vi "Facade_Create.vi"(0 "reference in":refnum<class "Facade.lvclass">, 2 "Home":refnum<class "House.lvclass">, 5 "Error In":errorcluster) -> (14 "reference out":refnum<class "Facade.lvclass">, 19 "Error Out":errorcluster)   [LabVIEW 2024, in "Facade.lvclass"]
uses:
  Facade.lvclass
  Facade.lvclass/Facade.ctl
  House/House_class/House.lvclass
panel:
  # "Connector Pane"
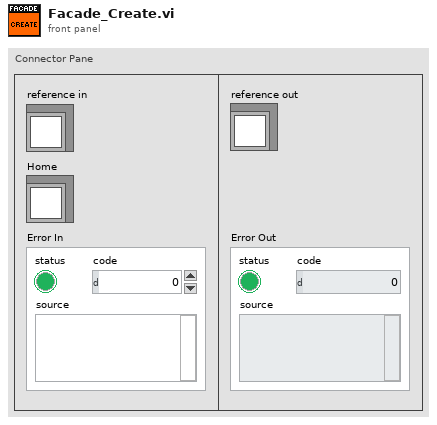
[diagram p1: front panel]
types:
  T1 = typedef "Facade.lvclass/ObjectAttributes.ctl" = cluster{"Home":refnum<class "House.lvclass">}
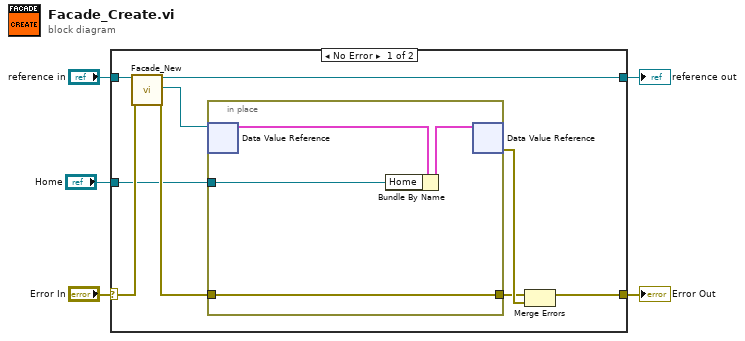
[diagram p0: block diagram]
diagram:
  n1 = case shown="No Error" "Error In" {
    selector: "Error In" -> [w13 w20]
    tunnel: [w10 w20] -> w4
    tunnel: "reference in" -> [w14 w19]
    tunnel: [w12 w19] -> w2
    tunnel: "Home" -> [w6 _]
    frame No Error {
      n2 = call "Facade_New.vi"("reference in"=w14, "Error In"=w13) -> ("reference out"=w12:refnum<class "Facade.lvclass">, "DVRRefOut"=w9:refnum<data-value>, "Error Out"=w8:errorcluster)  [unwired: 14 in, 1 out]
      n3 = in-place {
        in-place-border: w8 -> [w16]
        in-place-border: [w16] -> w7
        in-place-border: w6 -> [w15]
        n4 = in-place-dvr #1(w9) -> (w17:T1)  [unwired: 1 out]
        n5 = Bundle By Name(cluster=w17, "Home"=w15) -> (w18:T1)
        n6 = in-place-dvr #1(w18) -> (w11:errorcluster)  [unwired: 1 out]
      }
      n7 = Merge Errors(w7, w11) -> (w10:errorcluster)
    }
    frame Error {
      # "VI-TechBaseTemplate_Simple_6x8x6"
    }
  }
  "Error Out" <- w4
  "reference out" <- w2
